vi "startAutomatedTest.vi"(8 "error in (no error)":errorcluster, 10 "model":refnum<class "Model.lvclass">, 11 "InteractiveMotionState in":refnum<class "InteractiveSetpointState.lvclass">) -> (0 "error out":errorcluster, 2 "model 2":refnum<class "Model.lvclass">, 3 "InteractiveMotionState out":refnum<class "InteractiveSetpointState.lvclass">)   [LabVIEW 2013, in "InteractiveSetpointState.lvclass"]
uses:
  InteractiveSetpointState.lvclass
  Model/Model/Model.lvclass
  Typedefs/StateSelector.ctl
  Typedefs/FAMTTypedefs.lvlib
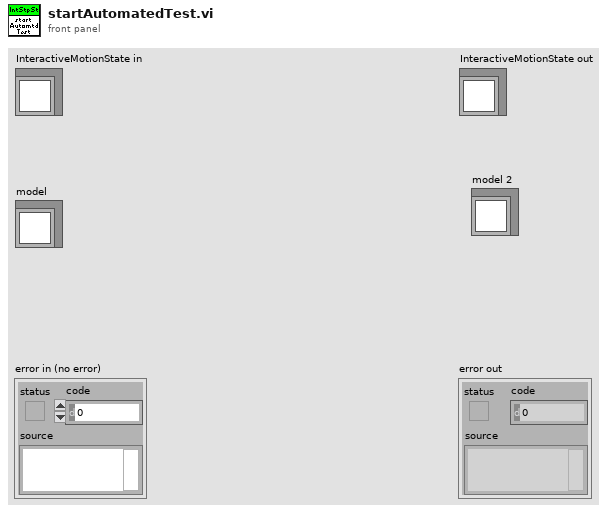
[diagram p1: front panel]
types:
  T1 = typedef "FAMTTypedefs.lvlib/StateSelector.ctl" = enum16{"EndingCycleState", "FaultState", "InteractiveSetpointState", "OffState", "StandbyState", "StoppedState"}
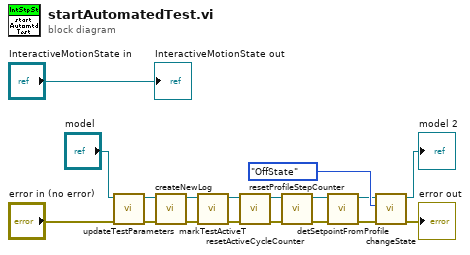
[diagram p0: block diagram]
diagram:
  n1 = call "updateTestParameters.vi"("error in (no error)"="error in (no error)", "Model in"="model") -> ("error out"=w7:errorcluster, "Model out"=w9:refnum<class "Model.lvclass">)  [unwired: 8 in]
  n2 = call "createNewLog.vi"("error in (no error)"=w7, "Model in"=w9) -> ("error out"=w12:errorcluster, "Model out"=w14:refnum<class "Model.lvclass">)  [unwired: 8 in]
  n3 = call "markTestActiveT.vi"("error in (no error)"=w12, "Model in"=w14) -> ("error out"=w11:errorcluster, "Model out"=w13:refnum<class "Model.lvclass">)  [unwired: 8 in]
  n4 = call "resetActiveCycleCounter.vi"("error in (no error)"=w11, "Model in"=w13) -> ("error out"=w3:errorcluster, "Model out"=w4:refnum<class "Model.lvclass">)  [unwired: 8 in]
  n5 = call "resetProfileStepCounter.vi"("error in (no error)"=w3, "Model in"=w4) -> ("error out"=w5:errorcluster, "Model out"=w6:refnum<class "Model.lvclass">)  [unwired: 8 in]
  n6 = call "detSetpointFromProfile.vi"("error in (no error)"=w5, "Model in"=w6) -> ("error out"=w1:errorcluster, "Model out"=w2:refnum<class "Model.lvclass">)  [unwired: 8 in]
  n7 = call "changeState.vi"("error in (no error)"=w1, "State:"=StateSelector."OffState", "Model in"=w2) -> ("error out"=→"error out":errorcluster, "Model out"=→"model 2":refnum<class "Model.lvclass">)  [unwired: 7 in]
  "InteractiveMotionState out" <- "InteractiveMotionState in"
